vi "Enqueue Open Connection.vi"(8 "Error In":errorcluster, 11 "Name":string) -> (0 "Error Out":errorcluster)   [LabVIEW 2019, in "Kolmogan Library 1.lvlib"]
uses:
  Kolmogan Library 1.lvlib
  Data Error Notifier/Data and Error Notifier.lvlib
  Queue/Queue.lvlib
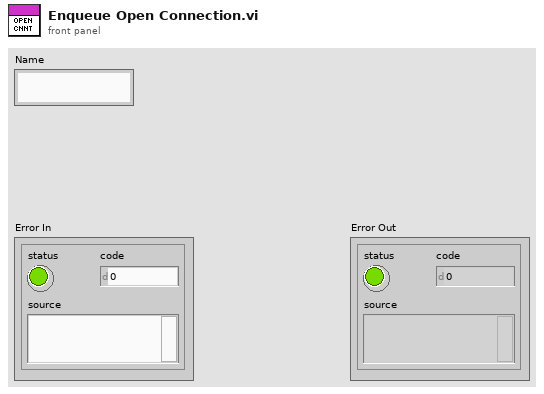
[diagram p1: front panel]
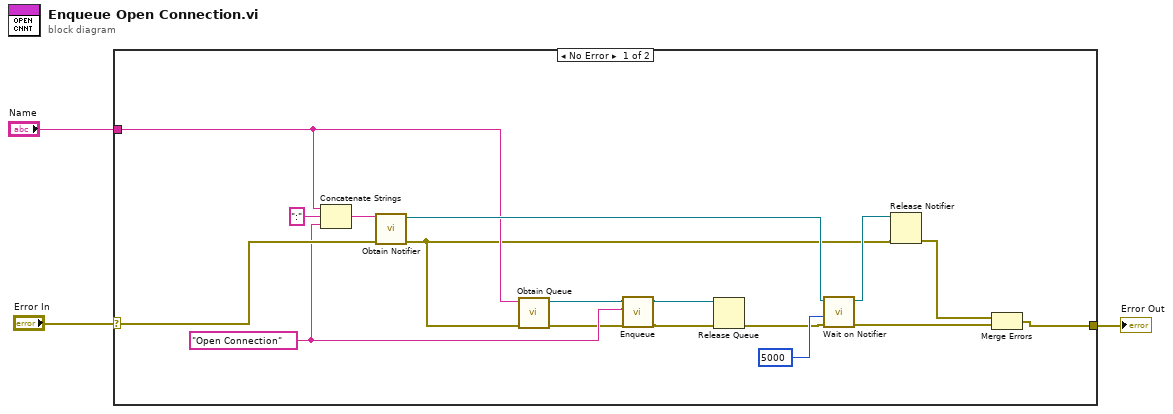
[diagram p0: block diagram]
diagram:
  n1 = case shown="No Error" "Error In" {
    selector: "Error In" -> [w16 w21]
    tunnel: [w18 w21] -> w2
    tunnel: "Name" -> [w10 _]
    frame No Error {
      w7 = "Open Connection" ("Message")
      n2 = Concatenate Strings(w10, ":" ("string"), w7) -> (w17:string)
      n3 = call "Obtain Notifier.vi"("Error In"=w16, "Name"=w17) -> ("Error Out"=w9:errorcluster, "notifier out"=w11:refnum<notifier>)  [unwired: 8 in]
      n4 = call "Obtain Queue.vi"("Error In"=w9, "Name"=w10) -> ("Error Out"=w4:errorcluster, "queue out"=w8:refnum<queue>)  [unwired: 8 in]
      n5 = call "Enqueue.vi"("Error In"=w4, "Message"=w7, "queue in"=w8) -> ("Error Out"=w6:errorcluster, "queue out"=w5:refnum<queue>)  [unwired: 7 in]
      n6 = Release Queue(queue=w5, error in (no error)=w6) -> (error out=w12:errorcluster)  [unwired: 1 in, 2 out]
      n7 = call "Wait on Notifier.vi"("Error In"=w12, "timeout in ms (-1)"=5000, "notifier in"=w11) -> ("Error Out"=w14:errorcluster, "notifier out"=w15:refnum<notifier>)  [unwired: 6 in, 1 out]
      n8 = Release Notifier(notifier=w15, error in (no error)=w9) -> (error out=w19:errorcluster)  [unwired: 1 in, 2 out]
      n9 = Merge Errors(w19, w14) -> (w18:errorcluster)
    }
    frame Error {
    }
  }
  "Error Out" <- w2
